vi "接收数据已改变回调VI.vi"(4 "Ctl引用句柄":refnum<vi>, 5 "事件数据":cluster{"sender":refnum<k24>, "e":refnum<k24>}, 6 "控件引用":refnum<k24>, 7 "事件通用数据":cluster{"事件源":i32, "事件类型":u32, "时间标识":u32}) -> ()   [LabVIEW 2012]
panel:
  out "ReadExisting":string
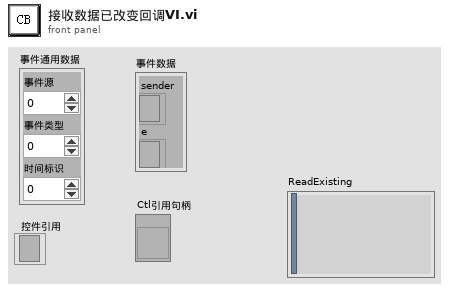
[diagram p1: front panel]
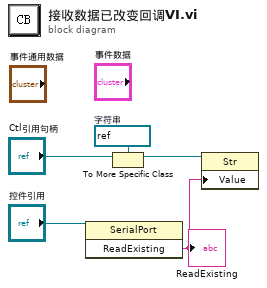
[diagram p0: block diagram]
diagram:
  w3 = refnum<vi> refnum  # 字符串
  n1 = invoke class="SerialPort" method="ReadExisting"(reference="控件引用") -> ("ReadExisting"=w1:string)  [unwired: 2 in, 2 out]
  "ReadExisting" <- w1
  n2 = To More Specific Class(target class=w3, reference="Ctl引用句柄") -> (specific class reference=w2:refnum<vi>)  [unwired: 1 in, 1 out]
  n3 = property class="Str"(reference=w2, "Value"=w1) -> ()  [unwired: 1 in, 2 out]
